vi "toTimestamp.vi"(7 "Use TAI Offset?":bool, 9 "Fractional Second":dbl format="%#.6f", 10 "UTC Time (s)":i64, 11 "Epoch (UTC)":refnum<class "Epoch.UTC.lvclass">) -> (1 "Not a Timestamp?":bool, 2 "Timestamp":timestamp, 3 "Epoch out":refnum<class "Epoch.UTC.lvclass">)   [LabVIEW 2018, in "Epoch.UTC.lvclass"]
uses:
  Epoch.UTC.lvclass
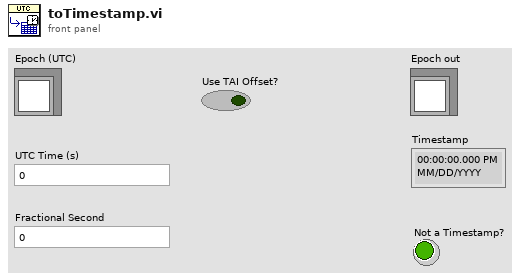
[diagram p1: front panel]
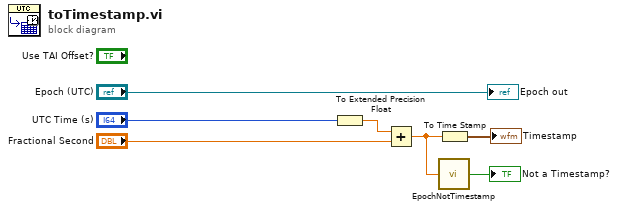
[diagram p0: block diagram]
diagram:
  n1 = To Extended Precision Float(1:"UTC Time (s)") -> (0:w7:ext)
  n2 = Add(x=w7, y="Fractional Second") -> (x+y=w4:ext)
  n3 = call "EpochNotTimestamp.vi"("Epoch Time"=w4) -> ("Not a Timestamp?"=→"Not a Timestamp?":bool)  [unwired: 8 in]
  n4 = To Time Stamp(1:w4) -> (0:→"Timestamp":timestamp)
  "Epoch out" <- "Epoch (UTC)"
